vi "initializePiece.vi"(8 "error in (no error)":errorcluster, 9 "startingSquare":string, 10 "pieceColor":T1, 11 "object in":refnum<class "Bishop.lvclass">) -> (0 "error out":errorcluster, 3 "object out":refnum<class "Bishop.lvclass">)   [LabVIEW 2020]
uses:
  Bishop.lvclass
  typedefs/pieceColor.ctl
  Piece.lvclass
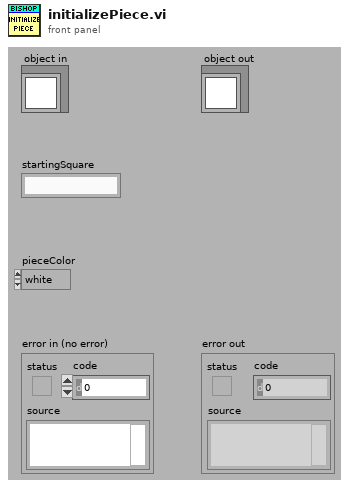
[diagram p1: front panel]
types:
  T1 = typedef "Piece.lvclass/pieceColor.ctl" = enum16{"white", "black"}
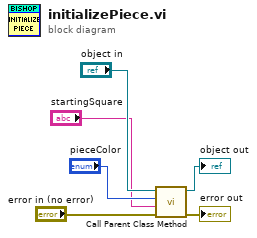
[diagram p0: block diagram]
diagram:
  n1 = call-parent "Call Parent Class Method"("error in (no error)"="error in (no error)", "startingSquare"="startingSquare", "pieceColor"="pieceColor", "object in"="object in") -> ("error out"=→"error out":errorcluster, "object out"=→"object out":refnum<class "Bishop.lvclass">)  [unwired: 6 in]
